vi "CamCache.vi"(6 "Shift":bool, 8 "Operation":enum16{"Set", "Get", "Wheel", "Drag"}(ring), 9 "Delta":i32, 10 "IncDrag":cluster{"X Cen":dbl, "Y Cen":dbl}, 11 "CamIn":T1) -> (3 "CamOut":T1)   [LabVIEW 2014]
uses:
  TypeDefs/Camera.ctl
  <vilib>/Utility/miscctls.llb/LV3DPointTypeDef.ctl
  <vilib>/Analysis/coordinate.llb/3D Coordinate Conversion (Scalar).vi
  <vilib>/Analysis/NI_AALPro.lvlib
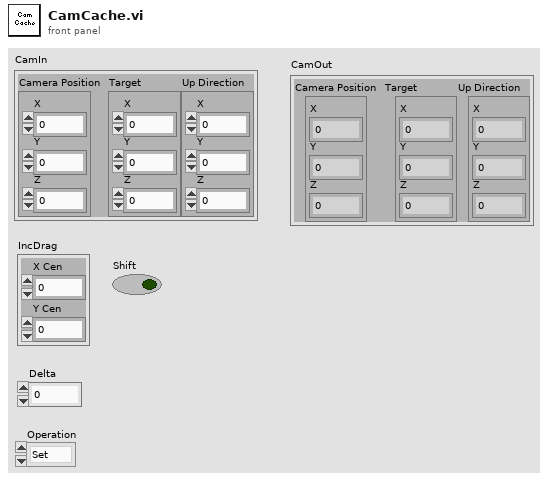
[diagram p1: front panel]
types:
  T1 = typedef "Camera.ctl" = cluster{"Camera Position":T2, "Target":T2, "Up Direction":T2}
  T2 = typedef "LV3DPointTypeDef.ctl" = cluster{"X":sgl, "Y":sgl, "Z":sgl}
  T3 = cluster{"axis 1 out":dbl, "axis 2 out":dbl, "axis 3 out":dbl}
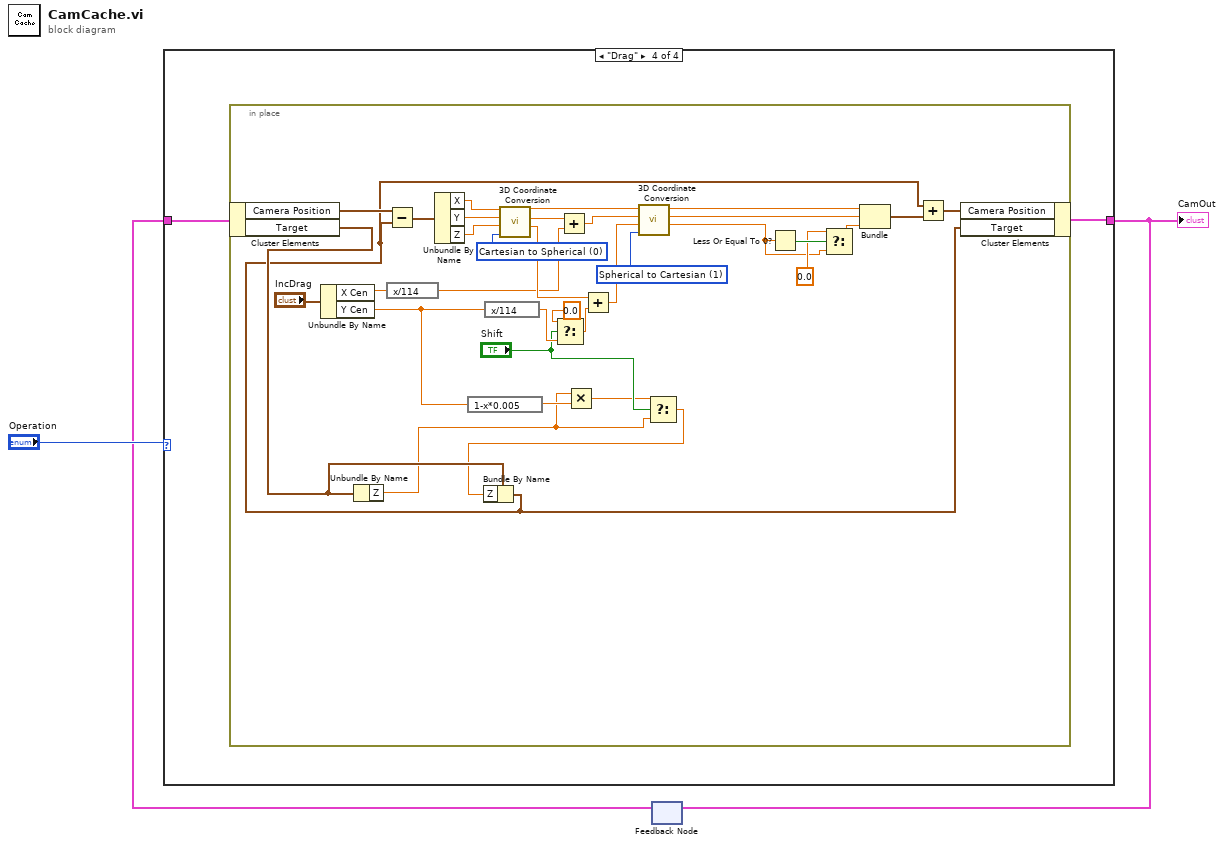
[diagram p0: block diagram]
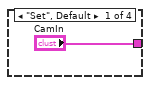
[diagram p2: hidden frame]
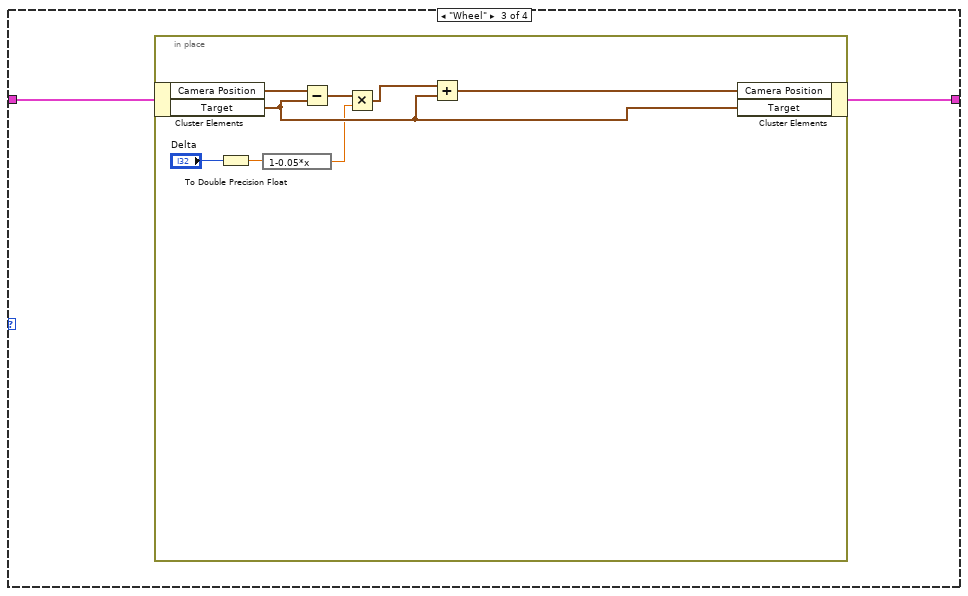
[diagram p4: hidden frame]
diagram:
  n1 = feedback #1() -> (w1:T1)  [unwired: 1 in]
  n2 = case shown="\"Drag\"" "Operation" {
    tunnel: ["CamIn" w5 w6 w16] -> w2
    tunnel: w1 -> [_ w5 w7 w17]
    frame "Set", Default {
    }
    frame "Get" {
    }
    frame "Wheel" {
      n3 = in-place {
        n4 = in-place-cluster #2(w7) -> ("Camera Position"=w14:T2, "Target"=w13:T2)
        n5 = To Double Precision Float(number="Delta") -> (double precision float=w8:dbl)
        n6 = expression code="1-0.05*x"(w8) -> (w12:dbl)
        n7 = Subtract(x=w14, y=w13) -> (x-y=w15:T2)
        n8 = Multiply(x=w15, y=w12) -> (x*y=w11:cluster{"X":dbl, "Y":dbl, "Z":dbl})
        n9 = Add(x=w11, y=w13) -> (x+y=w10:cluster{"X":dbl, "Y":dbl, "Z":dbl})
        n10 = in-place-cluster #2("Camera Position"=w10, "Target"=w13) -> (w6:T1)
      }
    }
    frame "Drag" {
      n11 = in-place {
        w34 = u16 1 items=["Cartesian to Spherical", "Spherical to Cartesian", "Cartesian to Cylindrical", "Cylindrical to Cartesian", "Spherical to Cylindrical", "Cylindrical to Spherical"] ("conversion type")
        w40 = u16 0 items=["Cartesian to Spherical", "Spherical to Cartesian", "Cartesian to Cylindrical", "Cylindrical to Cartesian", "Spherical to Cylindrical", "Cylindrical to Spherical"] ("conversion type")
        n12 = in-place-cluster #3(w17) -> ("Camera Position"=w51:T2, "Target"=w22:T2)
        n13 = Unbundle By Name("IncDrag") -> ("X Cen"=w48:dbl, "Y Cen"=w27:dbl)
        n14 = Unbundle By Name(w22) -> ("Z"=w19:sgl)
        n15 = expression code="x/114"(w48) -> (w31:dbl)
        n16 = expression code="1-x*0.005"(w27) -> (w26:dbl)
        n17 = expression code="x/114"(w27) -> (w29:dbl)
        n18 = Select(t=0.0, s="Shift", f=w29) -> (s? t:f=w30:dbl)
        n19 = Multiply(x=w19, y=w26) -> (x*y=w21:dbl)
        n20 = Select(t=w21, s="Shift", f=w19) -> (s? t:f=w20:dbl)
        n21 = Bundle By Name(cluster=w22, "Z"=w20) -> (w18:T2)
        n22 = Subtract(x=w51, y=w18) -> (x-y=w50:T2)
        n23 = Unbundle By Name(w50) -> ("X"=w42:sgl, "Y"=w41:sgl, "Z"=w25:sgl)
        n24 = call-poly <vilib>:"3D Coordinate Conversion.vi"("conversion type"=w40, "axis 3"=w25, "axis 2"=w41, "axis 1"=w42) -> ("axis 3 out"=w38:dbl, "axis 2 out"=w39:dbl, "axis 1 out"=w37:dbl)  [unwired: 4 in, 1 out]
        n25 = Add(x=w39, y=w31) -> (x+y=w36:dbl)
        n26 = Add(x=w38, y=w30) -> (x+y=w35:dbl)
        n27 = call-poly <vilib>:"3D Coordinate Conversion.vi"("conversion type"=w34, "axis 3"=w35, "axis 2"=w36, "axis 1"=w37) -> ("axis 3 out"=w23:dbl, "axis 2 out"=w32:dbl, "axis 1 out"=w33:dbl)  [unwired: 4 in, 1 out]
        n28 = Less Or Equal To 0?(x=w23) -> (x <= 0?=w45:bool)
        n29 = Select(t=0.0, s=w45, f=w23) -> (s? t:f=w44:dbl)
        n30 = Bundle("axis 1 out"=w33, "axis 2 out"=w32, "axis 3 out"=w44) -> (w47:T3)  [unwired: 1 in]
        n31 = Add(x=w18, y=w47) -> (x+y=w46:cluster{dbl, dbl, dbl})
        n32 = in-place-cluster #3("Camera Position"=w46, "Target"=w18) -> (w16:T1)
      }
    }
  }
  "CamOut" <- w2
  n33 = feedback-in #1(w2) -> ()
